vi "Ex1v3.vi"() -> ()   [LabVIEW 2017]
panel:
  in  "?":bool
  out "LED 5":bool
  out "LED 4":bool
  out "LED 3":bool
  out "LED2":bool
  out "LED1":bool
  in  "Délai":dbl(knob) scale=1.0..1000.0
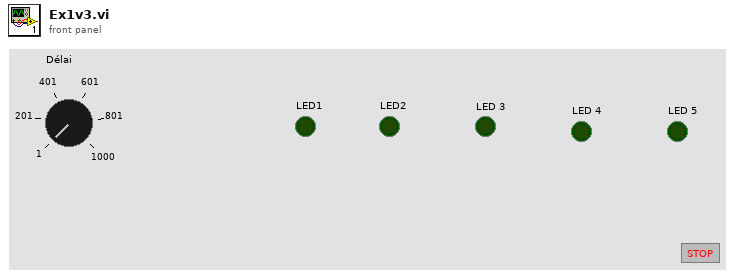
[diagram p1: front panel]
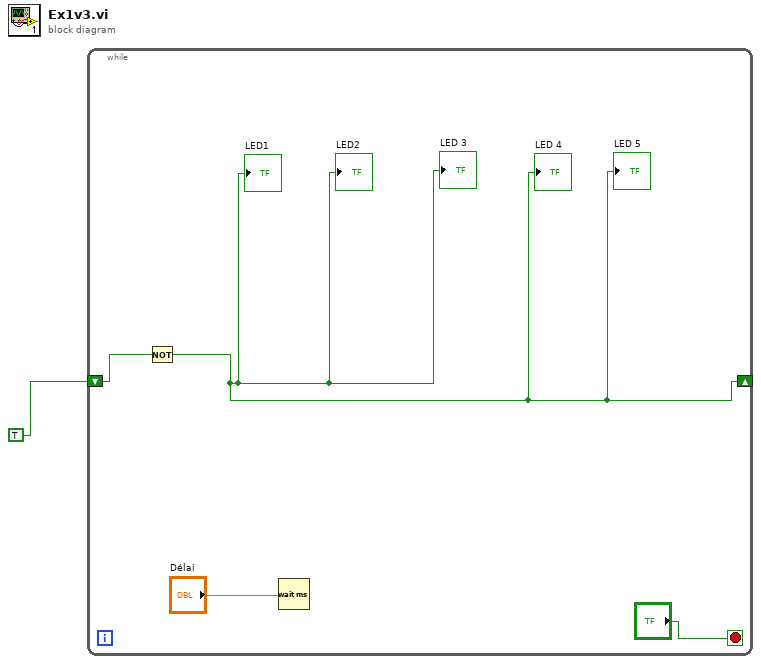
[diagram p0: block diagram]
diagram:
  n1 = while {
    shift-right: [w2] -> _
    shift-left: TRUE -> [w3]
    stop <- "?" stop-if-true
    n2 = Not(x=w3) -> (.not. x?=w2:bool)
    "LED1" <- w2
    "LED2" <- w2
    "LED 3" <- w2
    "LED 4" <- w2
    "LED 5" <- w2
    n3 = Wait (ms)(milliseconds to wait="Délai") -> ()  [unwired: 1 out]
  }
